vi "Globals.vi"() -> ()   [LabVIEW 2017, in "nifxpmath_DiscreteDelay.xnode"]
uses:
  <vilib>/rvi/FXPMathLib/basic elements/FxpDiscreteDelay/XNode/nifxpmath_DiscreteDelay.xnode
panel:
  in  "UPPER LIMIT OF WIDTH & DELAY":u32=512
  in  "TERM Addr NAME":string="n-1[0..%s]"
  in  "TERM Q NAME":string="Q"
  in  "TERM D NAME":string="D"
  in  "TERM Addr ID":string="TERM_ADDR"
  in  "TERM Q ID":string="TERM_Q"
  in  "TERM D ID":string="TERM_D"
  # "Width and delay number are limited to 512. We made this restriction to avoid causing the node slow. The limitation is used in both adaption to input and config dialog. Reasons for the value 512 are listed in CAR 202781 in more details."
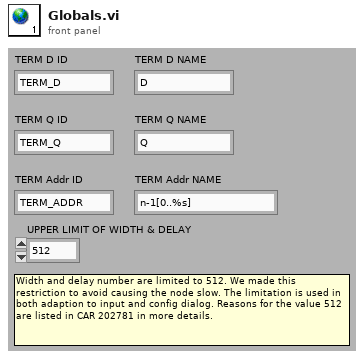
[diagram p1: front panel]
diagram:
